vi "Choose_cOPY.vi"(10 "Statuses":T1[](array[typedef]), 11 "Distances":dbl[](array[numeric])) -> (1 "distance of chosen book":dbl, 3 "status":T1)   [LabVIEW 2020]
uses:
  Controls/Book_Status.ctl
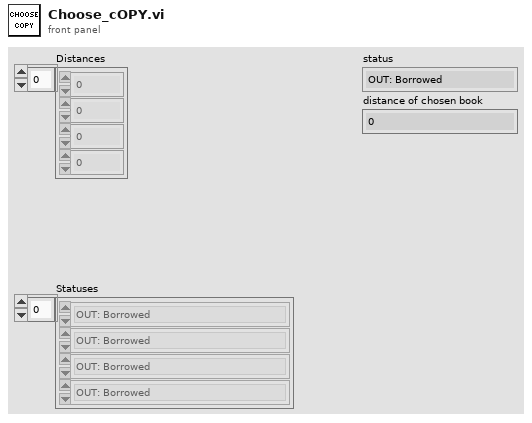
[diagram p1: front panel]
types:
  T1 = typedef "Book_Status.ctl" = enum16{"OUT: Borrowed", "OUT: In Segregation Machine", "IN: Currently In Use", "IN: Available", "IN: Misplaced", "IN: Location not found"}
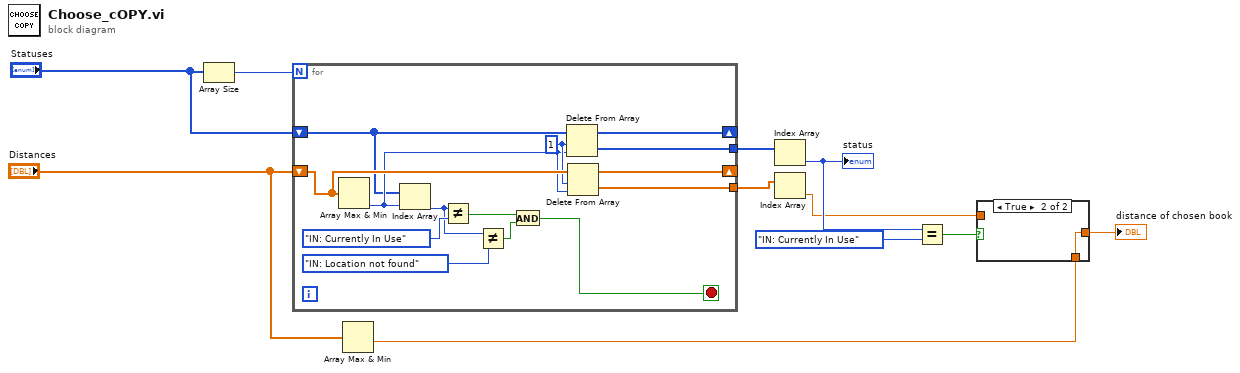
[diagram p0: block diagram]
diagram:
  n1 = Array Size(array="Statuses") -> (size(s)=w11:i32)
  n2 = for {
    N: w11 -> [_]
    tunnel: [w14] -> w9
    tunnel: [w13] -> w10
    shift-right: [w15] -> _
    shift-left: "Distances" -> [w18]
    shift-right: [w19] -> _
    shift-left: "Statuses" -> [w12]
    stop <- w20 stop-if-true
    w17 = 1 ("length")
    n3 = Array Max & Min(array=w18) -> (min index (indices)=w16:i32)  [unwired: 3 out]
    n4 = Index Array(array=w12, index=w16) -> (element=w24:T1)
    n5 = Not Equal?(x=w24, y=Book_Status."IN: Currently In Use") -> (x != y?=w21:bool)
    n6 = Not Equal?(x=w24, y=Book_Status."IN: Location not found") -> (x != y?=w22:bool)
    n7 = And(x=w21, y=w22) -> (x .and. y?=w20:bool)
    n8 = Delete From Array(array=w12, length=w17, index=w16) -> (deleted portion=w13:T1[], array with subset deleted=w19:T1[])
    n9 = Delete From Array(array=w18, length=w17, index=w16) -> (deleted portion=w14:dbl[], array with subset deleted=w15:dbl[])
  }
  n10 = Array Max & Min(array="Distances") -> (min value=w1:dbl)  [unwired: 3 out]
  n11 = Index Array(array=w10) -> (element=w6:T1)  [unwired: 1 in]
  "status" <- w6
  n12 = Index Array(array=w9) -> (element=w4:dbl)  [unwired: 1 in]
  n13 = Equal?(x=w6, y=Book_Status."IN: Currently In Use") -> (x = y?=w5:bool)
  n14 = case shown="True" w5 {
    tunnel: w4 -> [w26 _]
    tunnel: [w26 w27] -> w3
    tunnel: w1 -> [_ w27]
    frame False {
    }
    frame True {
    }
  }
  "distance of chosen book" <- w3
